vi "LOGclear_listeners.vi"(8 "Error In":errorcluster, 11 "Listeners In":T1[](array[typedef])) -> (0 "Error Out":errorcluster, 3 "Listeners Out":T1[](array[typedef]))   [LabVIEW 2025, in "LOGlib.lvlib"]
uses:
  LOGlog.ctl
  LOGstatement.ctl
  LOGtag.ctl
  LOGlib.lvlib
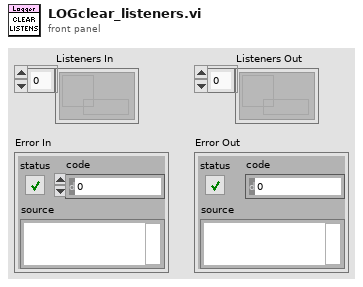
[diagram p1: front panel]
types:
  T1 = typedef "LOGlib.lvlib/LOGlog.ctl" = refnum<queue>
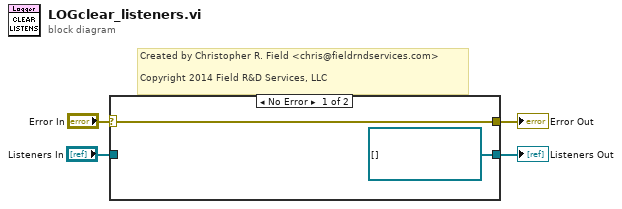
[diagram p0: block diagram]
diagram:
  # "Created by Christopher R. Field <chris@fieldrndservices.com>\n\nCopyright 2014 Field R&D Services, LLC"
  n1 = case shown="No Error" "Error In" {
    selector: "Error In" -> [w5 w7]
    tunnel: [T1[] [] w8] -> w4
    tunnel: "Listeners In" -> [_ w8]
    tunnel: [w5 w7] -> w1
    frame No Error {
    }
    frame Error {
    }
  }
  "Listeners Out" <- w4
  "Error Out" <- w1
